vi "PQsendPrepare.vi"(6 "paramTypes":u64, 7 "nParams":i64, 8 "error in (no error)":errorcluster, 9 "query":string, 10 "stmtName":string, 11 "conn":u64) -> (0 "error out":errorcluster, 2 "PQsendPrepare":i64, 3 "conn_out":u64)   [LabVIEW 2019, in "libpqlv64.lvlib"]
doc: "Sends a request to create a prepared statement with the given parameters, without waiting for completion.\n\n int PQsendPrepare(PGconn *conn,\n const char *stmtName,\n const char *query,\n int nParams,\n const Oid *paramTypes);\nThis is an asynchronous version of PQprepare\nhttp://www.postgresql.org/docs/8.3/static/libpq-async.html"
uses:
  libpqlv64.lvlib
  libpq.dll
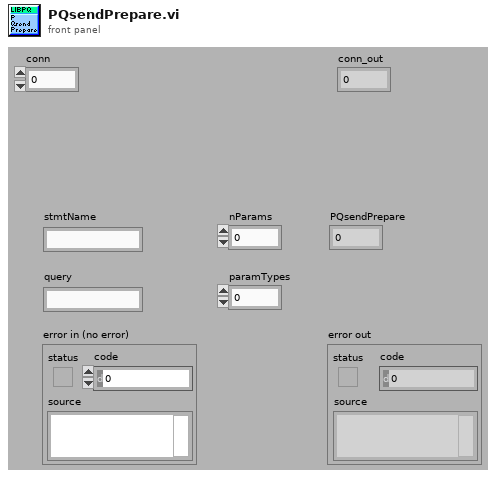
[diagram p1: front panel]
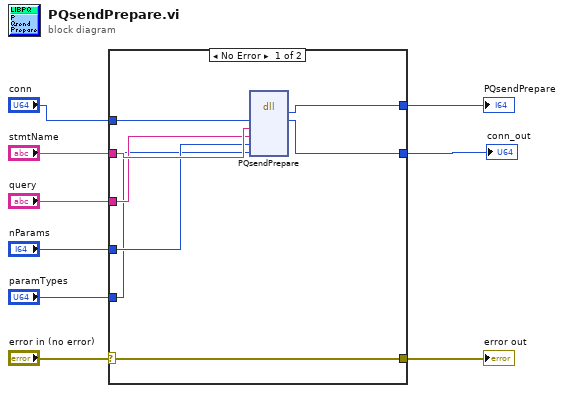
[diagram p0: block diagram]
diagram:
  n1 = case shown="No Error" "error in (no error)" {
    selector: "error in (no error)" -> [w17 w19]
    tunnel: [w17 w19] -> w8
    tunnel: [w16 _] -> w7
    tunnel: [w15 w18] -> w2
    tunnel: "stmtName" -> [w14 _]
    tunnel: "query" -> [w13 _]
    tunnel: "nParams" -> [w12 _]
    tunnel: "paramTypes" -> [w11 _]
    tunnel: "conn" -> [w10 w18]
    frame No Error {
      n2 = dll-call lib="libpq.*" fn="PQsendPrepare"("conn"=w10, "stmtName"=w14, "query"=w13, "nParams"=w12, "paramTypes"=w11) -> ("PQsendPrepare"=w16:i64, "conn"=w15:u64)  [unwired: 7 in, 2 out]
    }
    frame Error {
    }
  }
  "PQsendPrepare" <- w7
  "error out" <- w8
  "conn_out" <- w2
